vi "Sensor_Reference_Sensor.vi"() -> ()   [LabVIEW 2012]
doc: "This example VI demonstrates setting up a scan list and taking a reading using the advanced VIs. For more information about the different types of VIs, see the descriptions below.\n\nEven though only two types of measurements are shown, all six types can be configured in the same way. Likewise, this VI does not show every available configurable option for voltage and resistance.\n\n====================\nSetting up and performing a scan\n====================\nThe HP34970A provides commands for setting up a scan in three ways that differ in their complexity and the amount of control offered:\n\n1. Advanced:\nEvery aspect of the measurement, scan, scan list, and read is put in a different command to allow the greatest flexibility. For example, using the advanced configure VIs, you can set up a scan list consisting of different measurement types on different channels. The \"HP34970A Advanced Scan Example.vi\" demonstrates usage of these VIs.\n\n2. Medium:\nThe instrument also offers a command that wraps up configuring individual channels and the scan list. This is represented in the driver by \"HP34970A Conf EZ.vi\". This driver specifically replaces use of the advanced configure measurement VIs and configure scan list VIs. For more information, refer to the context help for the Conf EZ VI.\n\n3. Easiest:\nThe entire configuration, scan, and read are wrapped up into one command to the instrument. This is provided in this driver as the \"EZ\" VIs, which are in the Data subpalette of the HP34970A's driver palette. The \"HP34970A EZ Scan Example.vi\" demonstrates the EZ VI's usage."
uses:
  <instrlib>/Agilent 34970/Agilent 34970.lvlib
panel:
  in  "Numeric 2":i32=3
  in  "Numeric":i32=10
  in  "cancel measurement 2":bool
  in  "Advanced Config":T1={"Aperture Value (.4)"=0.4, "Aperture (1:Minimum)"=1, "NPLC (1)"=2, "Bandwidth (3 Hz)"=0, "Input Impedance (F:Fixed)"=FALSE, "Integration Time (F:Aperture)"=TRUE} {"Aperture (1:Minimum)" items=["Manual", "Minimum", "Maximum"]; "NPLC (1)" items=[".02", ".2", "1", "2", "10", "20", "100", "200", "Minimum", "Maximum"]; "Bandwidth (3 Hz)" items=["3 Hz", "20 Hz", "200 Hz", "Minimum", "Maximum"]}
  out "measuring time / ms":u32
  out "measurement running":bool
  in  "current transfer ratio":dbl[unit]=1.0 caption="s"
  in  "Sample interval":u32=100
  in  "cancel measurement":bool
  out "standard deviation / %":dbl=nan format="%#_3g"
  out "mean / V":dbl format="%0.2f"
  out "standard deviation / V":dbl format="%0.5f"
  out "Waveform Graph":T2(graph)={"Sample interval"=3, "Sample interval"=3, [0.0]}
  out "Readings":string[][](array[string])
  in  "Range (Volt.)":T3(ring)=enum."10 V"
  in  "Channel List (Volt.)":string="101"
  in  "VISA resource name":refnum<visa-resource-name>="USB0::0x0957::0x2007::MY49004365::INSTR"
  # "Voltage"
  # "target: 10ms stable"
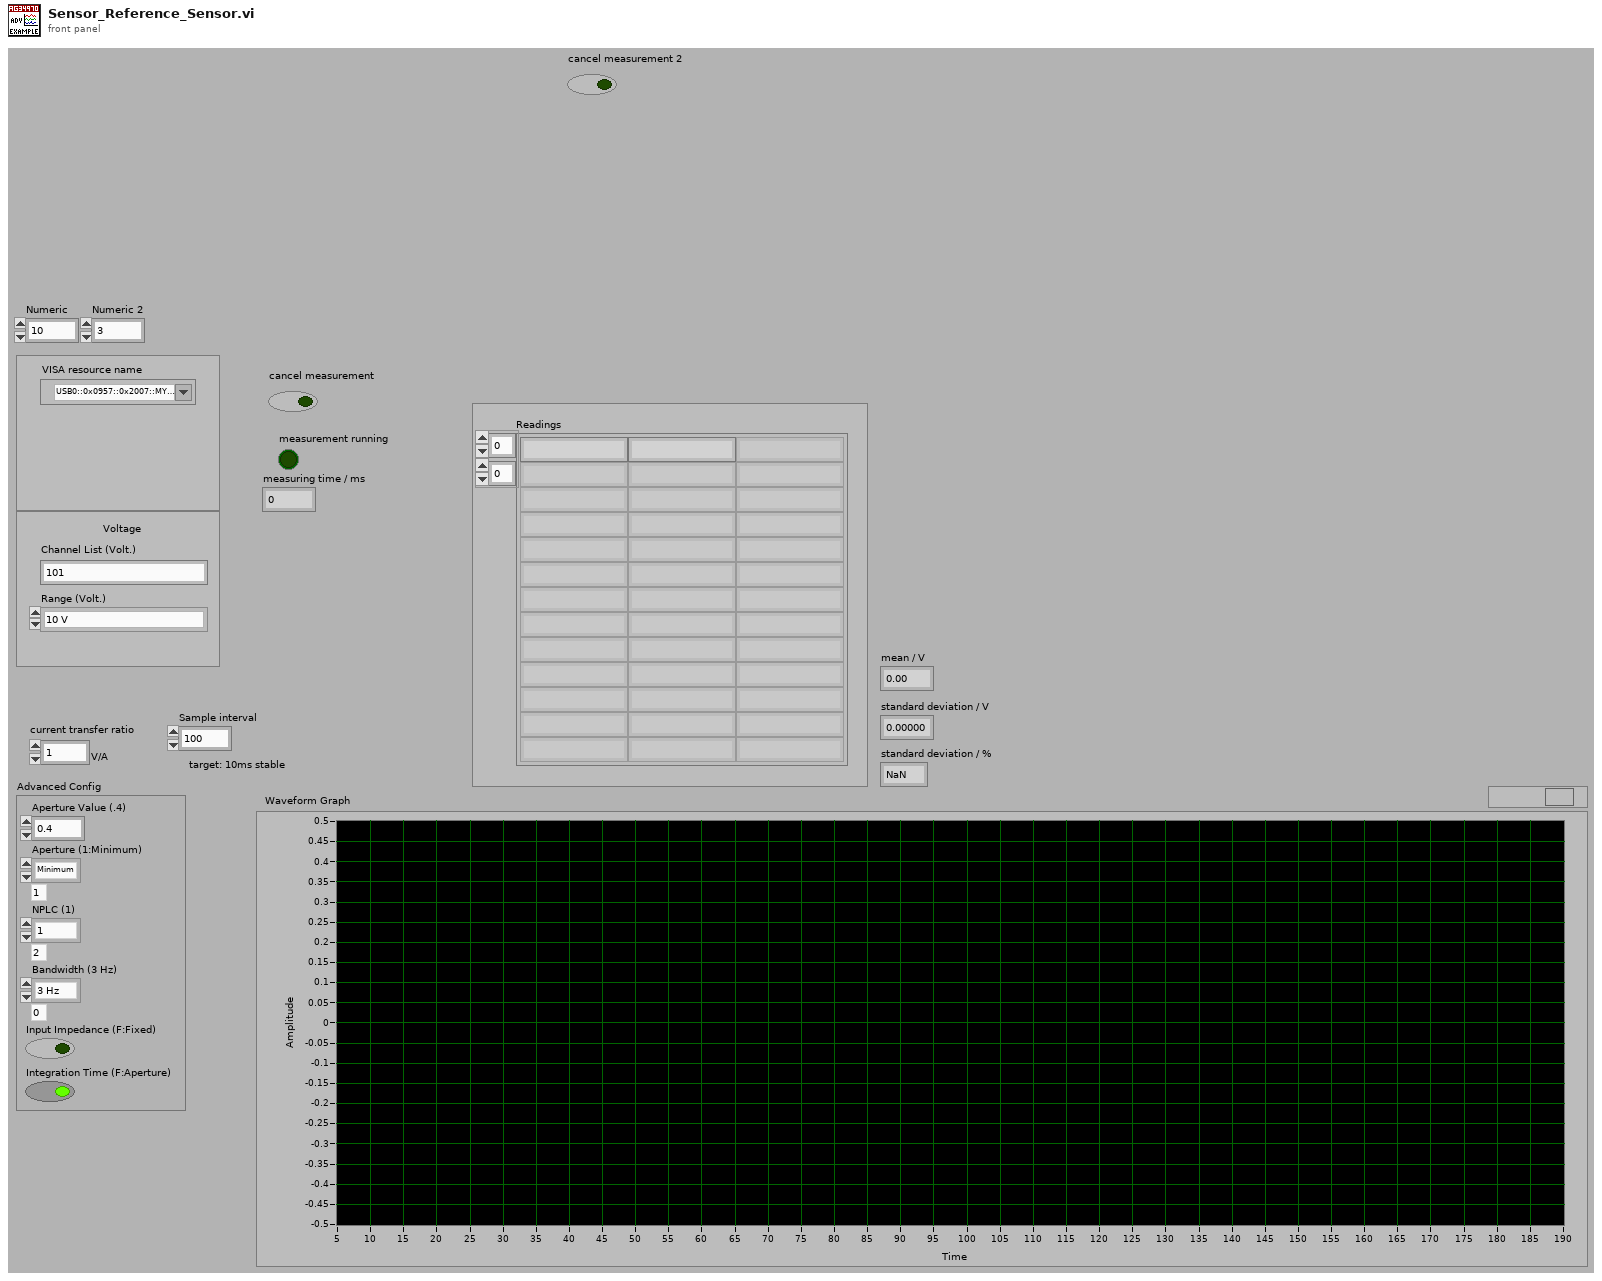
[diagram p1: front panel]
types:
  T1 = cluster{"Aperture Value (.4)":dbl, "Aperture (1:Minimum)":u16, "NPLC (1)":u16, "Bandwidth (3 Hz)":u16, "Input Impedance (F:Fixed)":bool, "Integration Time (F:Aperture)":bool}
  T2 = cluster{"Sample interval":u32, "Sample interval":u32, dbl[]}
  T3 = enum16{"100 mV", "1 V", "10 V", "100 V", "300 V", "Minimum", "Maximum"}
  T4 = cluster{"Include Alarm Data F:(No)":bool, "Include Channel # (F:No)":bool, "Include Time (F:No)":bool, "Include Units (F:No)":bool}
  T5 = enum16{"Bus", "Immediate", "External", "Alarm 1", "Alarm 2", "Alarm 3", "Alarm 4", "Timer"}
  T6 = cluster{"Timeout Value (10000)":u32, "Baud Rate (57600)":enum16{"1200", "2400", "4800", "9600", "19200", "38400", "57600", "115200"}, "Flow Control (1:XON/XOFF)":enum16{"None", "XON / XOFF", "RTS / CTS", "DTR / DSR"}}
  T7 = enum16{"Manual", "Minimum", "Maximum", "Infinity"}
  T8 = enum16{"Enable Register", "Event Register", "Operation Complete Bit"}
  T9 = enum16{"Remote Trigger", "Immediate Trigger", "Wait for Trigger", "Abort Scan"}
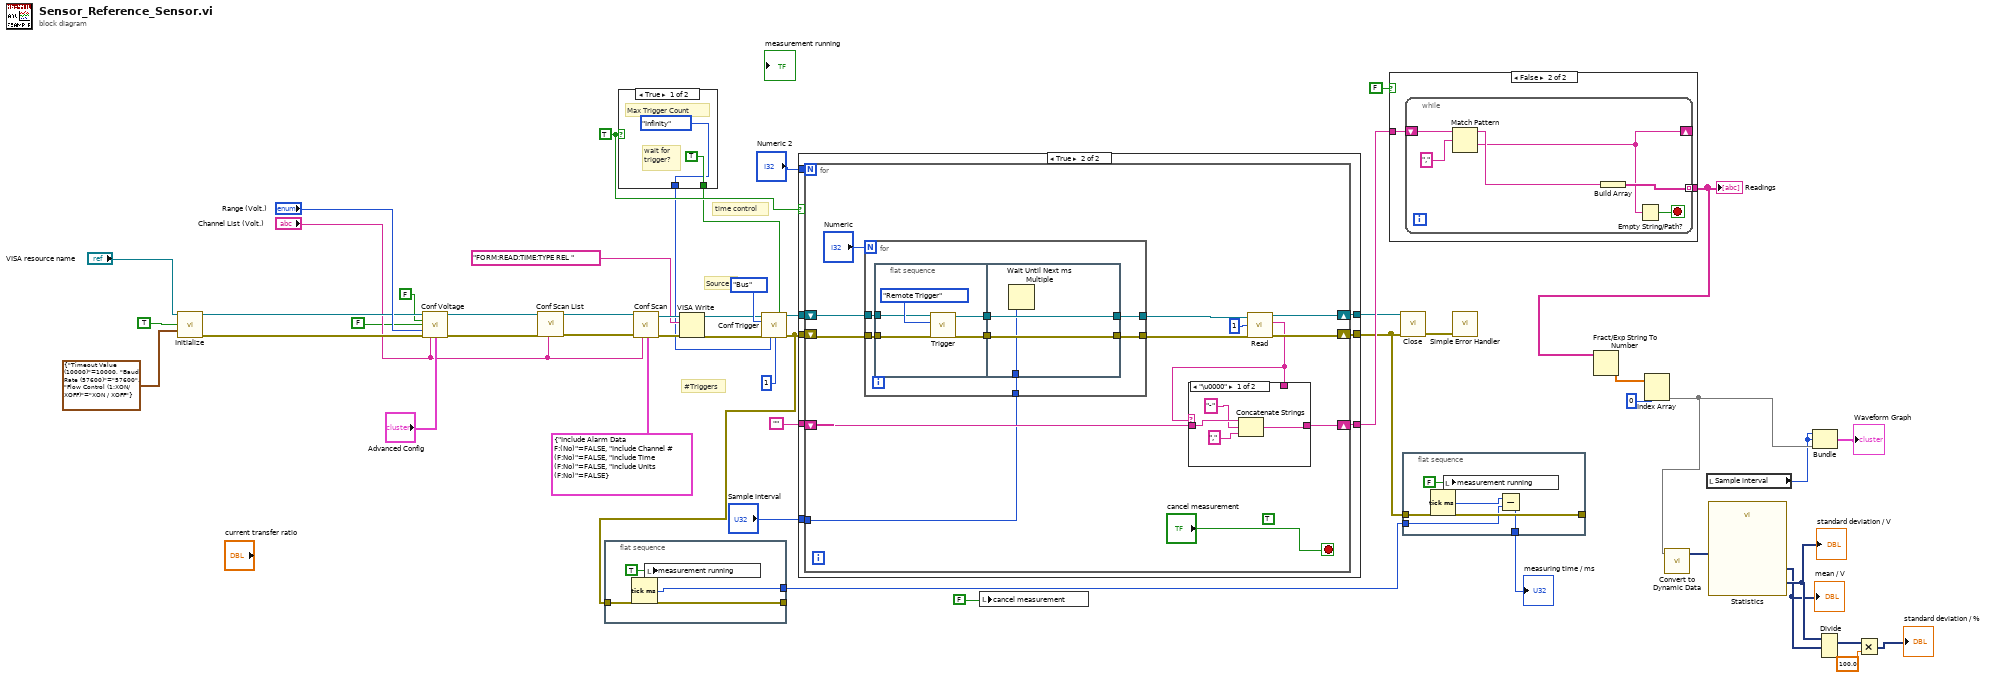
[diagram p0: block diagram]
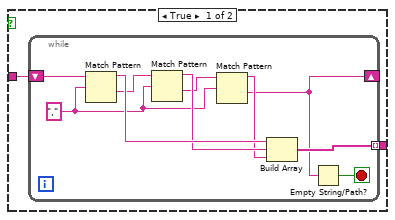
[diagram p2: hidden frame]
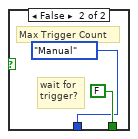
[diagram p3: hidden frame]
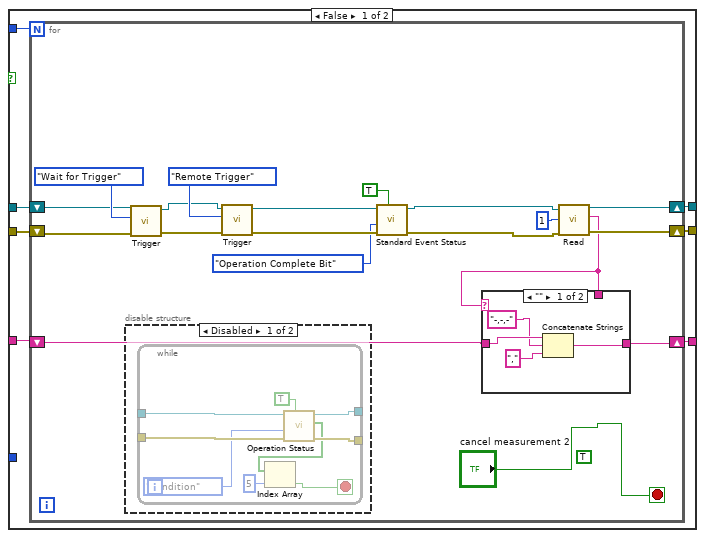
[diagram p4: hidden frame]
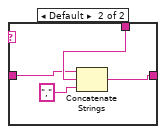
[diagram p5: hidden frame]
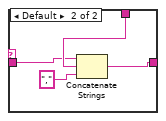
[diagram p7: hidden frame]
diagram:
  w4 = TRUE
  # "time control"
  # "Source"
  # "#Triggers"
  n1 = call <instrlib>:"Initialize.vi"("VISA Resource Name"="VISA resource name", "Reset (T: Reset)"=TRUE, "Serial Port Configuration"=T6 {"Timeout Value (10000)"=10000, "Baud Rate (57600)"=enum."57600", "Flow Control (1:XON/XOFF)"=enum."XON / XOFF"}) -> ("VISA Resource Name Out"=w47:refnum<visa-resource-name>, "error out"=w32:errorcluster)  [unwired: 11 in]
  n2 = call <instrlib>:"Conf Voltage.vi"("VISA Resource Name"=w47, "AC/DC (F:DC)"=FALSE, "Autorange? (F:Off)"=FALSE, "Range (6:Max)"="Range (Volt.)", "error in (no error)"=w32, "Channel List (empty)"="Channel List (Volt.)", "Advanced Config"="Advanced Config") -> ("VISA Resource Name Out"=w34:refnum<visa-resource-name>, "error out"=w25:errorcluster)  [unwired: 6 in, 1 out]
  n3 = call <instrlib>:"Conf Scan List.vi"("Scan List (empty)"="Channel List (Volt.)", "error in (no error)"=w25, "VISA Resource Name"=w34) -> ("error out"=w24:errorcluster, "VISA Resource Name Out"=w29:refnum<visa-resource-name>)  [unwired: 6 in, 1 out]
  n4 = flat-sequence {
    tunnel: w12 -> [w52]
    tunnel: [w52] -> _
    tunnel: [w51] -> w11
    frame #0 {
      n5 = Tick Count (ms)() -> (millisecond timer value=w51:u32)
      n6 = local write "measurement running"(TRUE ("measurement running")) -> ()
    }
  }
  n7 = case shown="True" w4 {
    tunnel: [TRUE ("Wait for Trigger? (F:No)") FALSE ("Wait for Trigger? (F:No)")] -> w3
    tunnel: [T7."Infinity" ("Max Trigger Count (3:Inf)") T7."Manual" ("Max Trigger Count (3:Inf)")] -> w2
    frame True {
      # "Max Trigger Count"
      # "wait for \ntrigger?"
    }
    frame False {
      # "Max Trigger Count"
      # "wait for \ntrigger?"
    }
  }
  n8 = call <instrlib>:"Conf Scan.vi"("VISA Resource Name"=w29, "error in (no error)"=w24, "Channel List (empty)"="Channel List (Volt.)", "Scan Fields"=T4 {"Include Alarm Data F:(No)"=FALSE, "Include Channel # (F:No)"=FALSE, "Include Time (F:No)"=FALSE, "Include Units (F:No)"=FALSE}) -> ("VISA Resource Name Out"=w9:refnum<visa-resource-name>, "error out"=w8:errorcluster)  [unwired: 9 in, 1 out]
  n9 = VISA Write(VISA resource name=w9, write buffer="FORM:READ:TIME:TYPE REL ", error in (no error)=w8) -> (VISA resource name out=w6:refnum<visa-resource-name>, error out=w7:errorcluster)  [unwired: 1 out]
  n10 = call <instrlib>:"Conf Trigger.vi"("VISA Resource Name"=w6, "Wait for Trigger? (F:No)"=w3, "Source (1:Immediate)"=T5."Bus", "error in (no error)"=w7, "Max Trigger Count (3:Inf)"=w2, "# Triggers (1)"=u16 1) -> ("VISA Resource Name Out"=w28:refnum<visa-resource-name>, "error out"=w12:errorcluster)  [unwired: 7 in, 1 out]
  n11 = case shown="True" w4 {
    tunnel: [w64 w108] -> w46
    tunnel: w28 -> [w61 w107]
    tunnel: "" -> [w59 w106]
    tunnel: "Sample interval" -> [_ w105]
    tunnel: [w62 w104] -> w16
    tunnel: "Numeric 2" -> [w58 w103]
    tunnel: [w63 w102] -> w13
    tunnel: w12 -> [w60 w101]
    frame False {
      n12 = for {
        N: w58 -> [_]
        shift-right: [w65] -> w64
        shift-left: w59 -> [w66]
        shift-right: [w82] -> w62
        shift-left: w61 -> [w76]
        shift-right: [w83] -> w63
        shift-left: w60 -> [w77]
        stop <- "cancel measurement 2" stop-if-true
        (unwired) TRUE
        n13 = disable-structure shown="Disabled" {
          frame Disabled {
            n14 = while {
              tunnel: _ -> [w100]
              tunnel: _ -> [w99]
              tunnel: [w96] -> _
              tunnel: [w95] -> _
              stop <- w92 stop-if-true
              n15 = call <instrlib>:"Operation Status.vi"("Set/Check (F:Set)"=TRUE, "error in (no error)"=w99, "Check Register(0:Condition)"=enum16{"Condition", "Enable", "Event"}."Condition", "VISA Resource Name"=w100) -> ("error out"=w95:errorcluster, "Bits Set"=w94:bool[], "VISA Resource Name Out"=w96:refnum<visa-resource-name>)  [unwired: 5 in]
              n16 = Index Array(array=w94, index=5) -> (element=w92:bool)
            }
          }
          frame Enabled {
          }
        }
        n17 = call <instrlib>:"Trigger.vi"("error in (no error)"=w77, "Command (0:Rem Trig)"=T9."Wait for Trigger", "VISA Resource Name"=w76) -> ("error out"=w74:errorcluster, "VISA Resource Name Out"=w75:refnum<visa-resource-name>)  [unwired: 7 in]
        n18 = call <instrlib>:"Trigger.vi"("error in (no error)"=w74, "Command (0:Rem Trig)"=T9."Remote Trigger", "VISA Resource Name"=w75) -> ("error out"=w71:errorcluster, "VISA Resource Name Out"=w72:refnum<visa-resource-name>)  [unwired: 7 in]
        n19 = call <instrlib>:"Standard Event Status.vi"("Set/Check? (F:Set)"=TRUE, "error in (no error)"=w71, "Check Parameter (0:Enable Reg)"=T8."Operation Complete Bit", "VISA Resource Name"=w72) -> ("error out"=w70:errorcluster, "VISA Resource Name Out"=w69:refnum<visa-resource-name>)  [unwired: 5 in, 1 out]
        n20 = call <instrlib>:"Read.vi"("error in (no error)"=w70, "# Channels (1)"=1 ("# Channels (0)"), "VISA Resource Name"=w69) -> ("error out"=w83:errorcluster, "Readings"=w67:string, "VISA Resource Name Out"=w82:refnum<visa-resource-name>)  [unwired: 5 in, 1 out]
        n21 = case shown="\"\"" w67 {
          tunnel: [w86 w91] -> w65
          tunnel: w67 -> [_ w90]
          tunnel: w66 -> [w85 w89]
          frame "" {
            n22 = Concatenate Strings(w85, "-,-,-" ("string"), "," ("string")) -> (w86:string)
          }
          frame Default {
            n23 = Concatenate Strings(w89, w90, "," ("string")) -> (w91:string)
          }
        }
      }
    }
    frame True {
      n24 = for {
        N: w103 -> [_]
        shift-right: [w120] -> w108
        shift-left: w106 -> [w119]
        tunnel: w105 -> [w113]
        shift-right: [w118] -> w104
        shift-left: w107 -> [w116]
        shift-right: [w121] -> w102
        shift-left: w101 -> [w115]
        stop <- "cancel measurement" stop-if-true
        (unwired) TRUE
        n25 = for {
          N: "Numeric" -> [_]
          tunnel: w116 -> [w126]
          tunnel: w115 -> [w125]
          tunnel: w113 -> [w124]
          tunnel: [w123] -> w112
          tunnel: [w122] -> w111
          n26 = flat-sequence {
            tunnel: w126 -> [w130]
            tunnel: w125 -> [w129]
            tunnel: [w132] -> w128
            tunnel: [w131] -> w127
            tunnel: [w135] -> w122
            tunnel: [w136] -> w123
            tunnel: w128 -> [w136]
            tunnel: w127 -> [w135]
            tunnel: w124 -> [w134]
            frame #0 {
              n27 = call <instrlib>:"Trigger.vi"("error in (no error)"=w129, "Command (0:Rem Trig)"=T9."Remote Trigger", "VISA Resource Name"=w130) -> ("error out"=w131:errorcluster, "VISA Resource Name Out"=w132:refnum<visa-resource-name>)  [unwired: 7 in]
            }
            frame #1 {
              n28 = Wait Until Next ms Multiple(millisecond multiple=w134) -> ()  [unwired: 1 out]
            }
          }
        }
        n29 = call <instrlib>:"Read.vi"("error in (no error)"=w111, "# Channels (1)"=1 ("# Channels (0)"), "VISA Resource Name"=w112) -> ("error out"=w121:errorcluster, "Readings"=w110:string, "VISA Resource Name Out"=w118:refnum<visa-resource-name>)  [unwired: 5 in, 1 out]
        n30 = case shown="\"\"" w110 {
          tunnel: [w139 w144] -> w120
          tunnel: w110 -> [_ w143]
          tunnel: w119 -> [w138 w142]
          frame "\u0000" {
            n31 = Concatenate Strings(w138, "-" ("string"), "," ("string")) -> (w139:string)
          }
          frame Default {
            n32 = Concatenate Strings(w142, w143, "," ("string")) -> (w144:string)
          }
        }
      }
    }
  }
  n33 = local write "cancel measurement"(FALSE ("Boolean")) -> ()
  n34 = case shown="False" FALSE {
    tunnel: w46 -> [w146 w158]
    tunnel: [w145 w157] -> w44
    frame True {
      n35 = while {
        tunnel: [w153] -> w145 mode=indexing
        shift-left: w146 -> [w156]
        shift-right: [w148] -> _
        stop <- w152 stop-if-true
        w147 = "," ("regular expression")
        n36 = Match Pattern(string=w156, regular expression=w147) -> (before substring=w155:string, after substring=w151:string)  [unwired: 1 in, 2 out]
        n37 = Match Pattern(string=w151, regular expression=w147) -> (before substring=w154:string, after substring=w150:string)  [unwired: 1 in, 2 out]
        n38 = Match Pattern(string=w150, regular expression=w147) -> (before substring=w149:string, after substring=w148:string)  [unwired: 1 in, 2 out]
        n39 = Build Array(w155, w154, w149) -> (w153:string[])
        n40 = Empty String/Path?(string/path=w148) -> (empty?=w152:bool)
      }
    }
    frame False {
      n41 = while {
        tunnel: [w162] -> w157 mode=indexing
        shift-left: w158 -> [w164]
        shift-right: [w159] -> _
        stop <- w161 stop-if-true
        n42 = Match Pattern(string=w164, regular expression=",") -> (before substring=w163:string, after substring=w159:string)  [unwired: 1 in, 2 out]
        n43 = Build Array(w163) -> (w162:string[])
        n44 = Empty String/Path?(string/path=w159) -> (empty?=w161:bool)
      }
    }
  }
  "Readings" <- w44
  n45 = call <instrlib>:"Close.vi"("VISA Resource Name"=w16, "error in (no error)"=w13) -> ("error out"=w49:errorcluster)  [unwired: 13 in]
  n46 = flat-sequence {
    tunnel: w13 -> [w168]
    tunnel: [w168] -> _
    tunnel: w11 -> [w166]
    tunnel: [w165] -> w10
    frame #0 {
      n47 = Tick Count (ms)() -> (millisecond timer value=w167:u32)
      n48 = local write "measurement running"(FALSE ("measurement running")) -> ()
      n49 = Subtract(x=w167, y=w166) -> (x-y=w165:u32)
    }
  }
  n50 = call <vilib>:"Simple Error Handler.vi"("error in (no error)"=w49) -> ()  [unwired: 4 in, 5 out]
  n51 = Fract/Exp String To Number(string=w44) -> (number=w43:dbl[][])  [unwired: 3 in, 1 out]
  n52 = Index Array(array=w43, index (col)=0 ("disabled index (col)")) -> (element=w35:dbl[])  [unwired: 1 in]
  n53 = call "Convert to Dynamic Data"("Array"=w35) -> ("Dynamic Data Type"=w41:dynamicdata)  [unwired: 3 in]
  n54 = local read "Sample interval"() -> (w23:u32)
  n55 = call "Statistics"("Signals"=w41) -> ("Standard Dev"=w40:dynamicdata, "Arithmetic Mean"=w39:dynamicdata)  [unwired: 24 in, 1 out]
  "standard deviation / V" <- w40
  "mean / V" <- w39
  n56 = Bundle("Sample interval"=w23, "Sample interval"=w23, w35) -> (→"Waveform Graph":T2)  [unwired: 1 in]
  n57 = Divide(1:w39, 2:w40) -> (0:w38:dynamicdata)  [unwired: 1 in, 1 out]
  n58 = Multiply(x=w38, y=100.0) -> (x*y=→"standard deviation / %":dynamicdata)
  "measuring time / ms" <- w10
